vi "Credentials.vi"(0 "Path":path, 1 "Device Name":string, 3 "error in (no error)":errorcluster) -> (7 "Cluster":T1, 9 "Found":bool, 10 "error out":errorcluster)   [LabVIEW 2013, in "IOTFoundation.lvlib"]
uses:
  <vilib>/Utility/config.llb/Read Key (String).vi
  IOTFoundation.lvlib
  <vilib>/Utility/config.llb/NI_LVConfig.lvlib
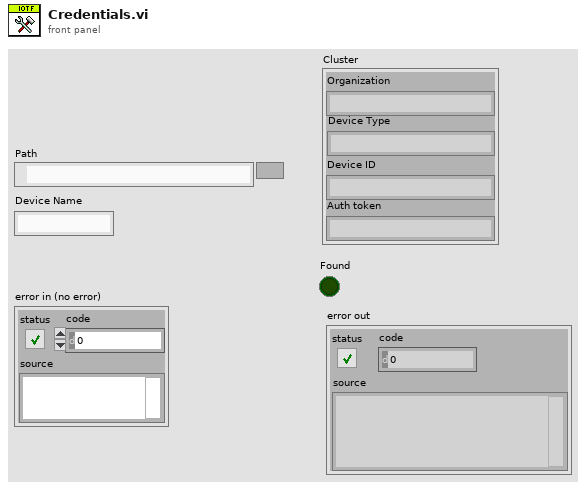
[diagram p1: front panel]
types:
  T1 = cluster{"Organization":string, "Device Type":string, "Device ID":string, "Auth token":string}
  T2 = typedef "NI_LVConfig.lvlib/Config Data RefNum.ctl" = refnum<k1>
  T3 = cluster{"value":string, "value":string, "value":string, "value":string}
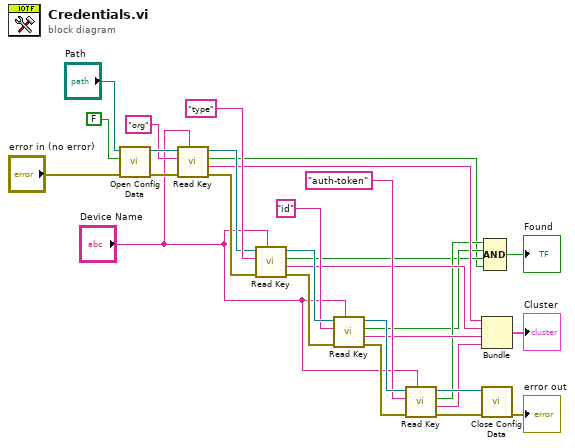
[diagram p0: block diagram]
diagram:
  n1 = call <vilib>:"Open Config Data.vi"("error in (no error)"="error in (no error)", "create file if necessary (T)"=FALSE, "configuration file path"="Path") -> ("error out"=w28:errorcluster, "refnum"=w29:T2)  [unwired: 6 in, 1 out]
  n2 = call-poly <vilib>:"Read Key.vi"("section"="Device Name", "error in (no error)"=w28, "key"="org", "refnum"=w29) -> ("error out"=w23:errorcluster, "value"=w14:string, "found?"=w4:bool, "refnum out"=w24:T2)  [unwired: 4 in]
  n3 = call-poly <vilib>:"Read Key.vi"("section"="Device Name", "error in (no error)"=w23, "key"="type", "refnum"=w24) -> ("error out"=w20:errorcluster, "value"=w13:string, "found?"=w5:bool, "refnum out"=w22:T2)  [unwired: 4 in]
  n4 = call-poly <vilib>:"Read Key.vi"("section"="Device Name", "error in (no error)"=w20, "key"="id", "refnum"=w22) -> ("error out"=w19:errorcluster, "value"=w12:string, "found?"=w6:bool, "refnum out"=w18:T2)  [unwired: 4 in]
  n5 = call-poly <vilib>:"Read Key.vi"("section"="Device Name", "error in (no error)"=w19, "key"="auth-token", "refnum"=w18) -> ("error out"=w16:errorcluster, "value"=w11:string, "found?"=w7:bool, "refnum out"=w15:T2)  [unwired: 4 in]
  n6 = Bundle("value"=w14, "value"=w13, "value"=w12, "value"=w11) -> (→"Cluster":T3)  [unwired: 1 in]
  n7 = call <vilib>:"Close Config Data.vi"("error in (no error)"=w16, "refnum"=w15) -> ("error out"=→"error out":errorcluster)  [unwired: 8 in, 1 out]
  n8 = Compound Arithmetic op=AND(w7, w6, w5, w4) -> (→"Found":bool)
